vi "Asynchronous Call.vi"() -> ()   [LabVIEW 2020]
panel:
  out "TimeStamp":timestamp
  in  "delayInSeconds":dbl=2.5
  in  "stop":bool
  out "iterations":i32
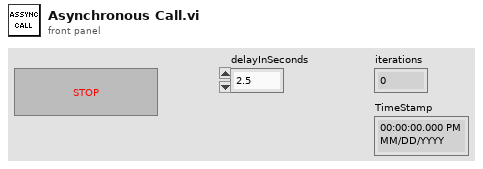
[diagram p1: front panel]
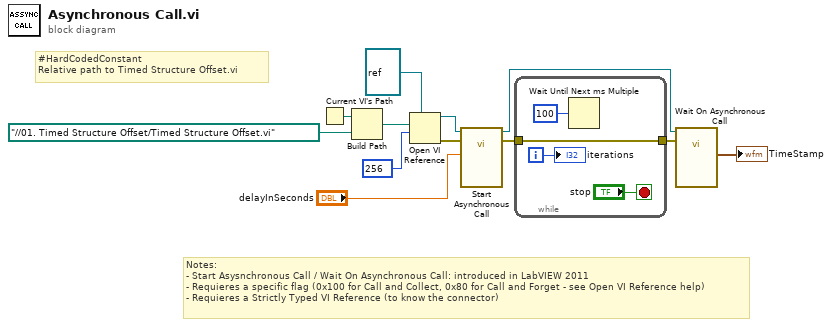
[diagram p0: block diagram]
diagram:
  # "#HardCodedConstant\nRelative path to Timed Structure Offset.vi"
  # "Notes:\n- Start Asysnchronous Call / Wait On Asynchronous Call: introduced in LabVIEW 2011\n- Requieres a specific flag (0x100 for Call and Collect, 0x80 for Call and Forget - see Open VI Reference help)\n- Requieres a Strictly Typed VI Reference (to know the connector)"
  n1 = Current VI's Path() -> (path=w3:path)
  n2 = Build Path(base path=w3, name or relative path=path "../../01. Timed Structure Offset/Timed Structure Offset.vi") -> (appended path=w1:path)
  n3 = Open VI Reference(type specifier VI Refnum (for type only)=refnum<vi> refnum, vi path=w1, options=256) -> (vi reference=w12:refnum<vi>, error out=w11:errorcluster)  [unwired: 3 in]
  n4 = call-by-ref "Start Asynchronous Call"(reference=w12, error in=w11, "delayInSeconds"="delayInSeconds") -> (reference out=w7:refnum<vi>, error out=w8:errorcluster)  [unwired: 10 in, 1 out]
  n5 = while {
    tunnel: w8 -> [w13]
    tunnel: [w13] -> w6
    i -> [w16]
    stop <- "stop" stop-if-true
    n6 = Wait Until Next ms Multiple(millisecond multiple=u32 100) -> ()  [unwired: 1 out]
    "iterations" <- w16
  }
  n7 = call-by-ref "Wait On Asynchronous Call"(reference=w7, error in=w6) -> ("TimeStamp"=→"TimeStamp":timestamp)  [unwired: 11 in, 2 out]
